vi "sender.vi"() -> ()   [LabVIEW 2013]
uses:
  <vilib>/sound2/lvsound2.llb/Sound Data Format.ctl
  <vilib>/sound2/lvsound2.llb/Sampling Mode.ctl
  <vilib>/sound2/lvsound2.llb/Sound Output Set Volume (Single).vi
  <vilib>/sound2/lvsound2.llb/Sound Output Write (DBL Single).vi
  <vilib>/express/express analysis/Spectral/Block/exnSpectralBlock spectral measurements RMS poly.vi
  <vilib>/express/express analysis/Spectral/Block/exnSpectralBlock spectral measurements RMS WFM.vi
  <vilib>/express/express analysis/Spectral/XNode/ExpressSpectralMeasurementsBlockNode.xnode
panel:
  in  "period(s)":dbl
  in  "index":i32
  in  "volume":dbl=100.0
  in  "device ID":u32
  out "Waveform Graph":cluster{"f0":dbl, "df":dbl, "magnitude":dbl[]}(graph)
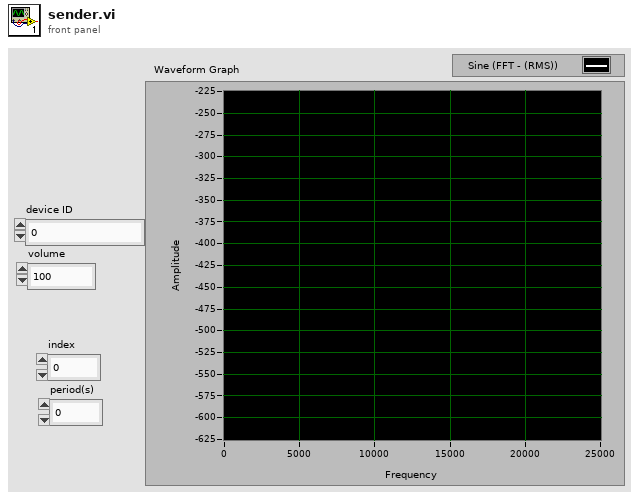
[diagram p1: front panel]
types:
  T1 = typedef "Sampling Mode.ctl" = i32
  T2 = typedef "Sound Data Format.ctl" = cluster{"sample rate (S/s)":dbl, "number of channels":i32, "bits per sample":i32}
  T3 = typedef "Sound Output Task ID.ctl" = u32
  T4 = cluster{"averaging mode":u16, "weighting mode":u16, "number of averages":u32}
  T5 = cluster{"dB On (F)":bool, "unwrap phase (F)":bool, "convert to degree (F)":bool}
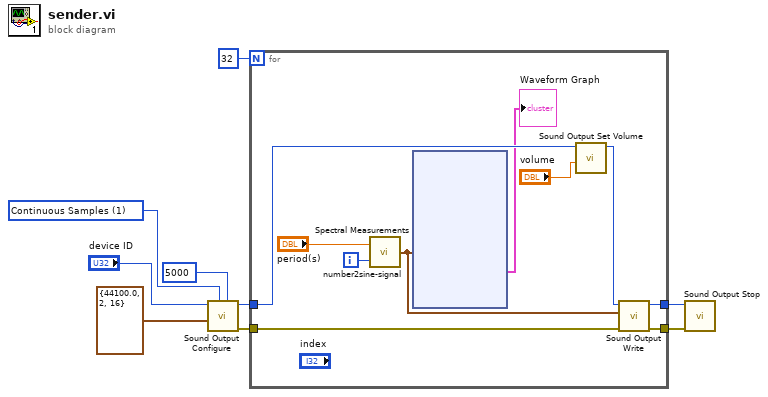
[diagram p0: block diagram]
diagram:
  w6 = T1 1 items=["Finite Samples", "Continuous Samples"] ("sample mode")
  n1 = call <vilib>:"Sound Output Configure.vi"("number of samples/ch"=5000, "sample mode"=w6, "sound format"=T2 {"sample rate (S/s)"=44100.0, "number of channels"=2, "bits per sample"=16}, "device ID"="device ID") -> ("error out"=w2:errorcluster, "task ID"=w4:T3)  [unwired: 6 in]
  n2 = for {
    N: 32 -> [_]
    tunnel: [w19] -> w9
    tunnel: w4 -> [w17]
    tunnel: w2 -> [w15]
    tunnel: [w14] -> w3
    i -> [w10]
    n3 = call "number2sine-signal.vi"("index(0~31)"=w10, "period(s)"="period(s)") -> ("signal out"=w11:waveform(dbl))  [unwired: 1 in]
    n4 = xnode "Spectral Measurements"("Signals"=w11) -> ("FFT - (RMS)"=→"Waveform Graph":cluster{"f0":dbl, "df":dbl, "magnitude":dbl[]})  [unwired: 1 in, 2 out]
    n5 = call-poly <vilib>:"Sound Output Set Volume.vi"("volume"="volume", "task ID"=w17) -> ("task ID out"=w18:T3)  [unwired: 8 in, 1 out]
    n6 = call-poly <vilib>:"Sound Output Write.vi"("error in (no error)"=w15, "data"=w11, "task ID"=w18) -> ("error out"=w14:errorcluster, "task ID out"=w19:T3)  [unwired: 7 in]
  }
  n7 = call <vilib>:"Sound Output Stop.vi"("error in (no error)"=w3, "task ID"=w9) -> ()  [unwired: 8 in, 2 out]
